vi "Main_ProducerConsumer.vi"() -> ()   [LabVIEW 2014]
doc: "Use this template to build a producer/consumer design pattern. Use this template when you need to execute a process, such as data analysis, when a data source, such as a triggered acquisition, produces data at an uneven rate and you need to execute the process when the data becomes available."
panel:
  in  "WebApp Sensor Data":T1
  in  "WebApp Plug Data":T2
  in  "WebApp Sensors":T3
  in  "WebApp Plugs":T4
  out "plug5option":string
  out "plug4option":string
  out "plug3option":string
  out "plug2option":string
  out "plug1option":string
  out "humidity":string
  out "luminosity":string
  out "temperature":string
  out "Outlet5_Output":bool
  in  "Outlet5_Input":bool
  out "Outlet4_Output":bool
  in  "Outlet4_Input":bool
  out "Outlet3_Output":bool
  in  "Outlet3_Input":bool
  out "Outlet2_Output":bool
  in  "Outlet2_Input":bool
  out "Outlet1_Output":bool
  in  "Outlet1_Input":bool
  in  "Outlet5_Refnum":refnum<k21>="ni.var.psp://Deepak-PC/Shared Variable Library Master/Outlet5"
  in  "Outlet4_Refnum":refnum<k21>="ni.var.psp://Deepak-PC/Shared Variable Library Master/Outlet4"
  in  "Outlet3_Refnum":refnum<k21>="ni.var.psp://Deepak-PC/Shared Variable Library Master/Outlet3"
  in  "Outlet2_Refnum":refnum<k21>="ni.var.psp://Deepak-PC/Shared Variable Library Master/Outlet2"
  in  "Outlet1_Refnum":refnum<k21>="ni.var.psp://Deepak-PC/Shared Variable Library Master/Outlet1"
  in  "stop":bool
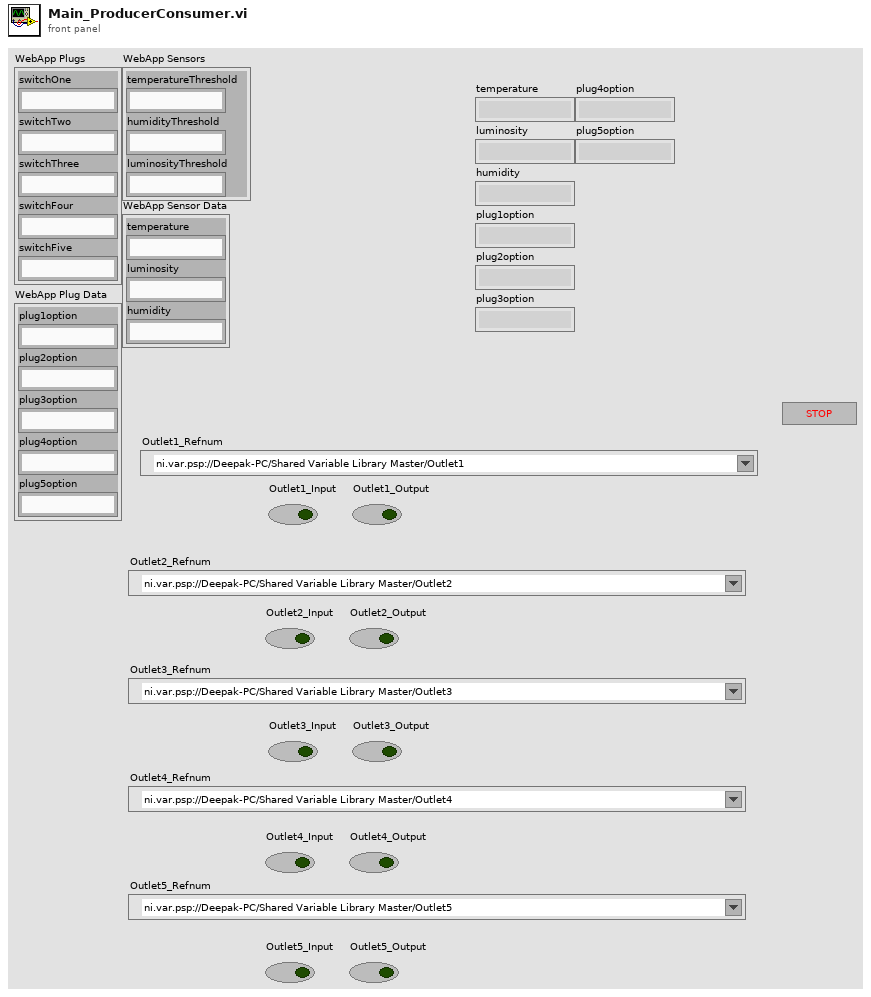
[diagram p1: front panel]
types:
  T1 = cluster{"temperature":string, "luminosity":string, "humidity":string}
  T2 = cluster{"plug1option":string, "plug2option":string, "plug3option":string, "plug4option":string, "plug5option":string}
  T3 = cluster{"temperatureThreshold":string, "humidityThreshold":string, "luminosityThreshold":string}
  T4 = cluster{"switchOne":string, "switchTwo":string, "switchThree":string, "switchFour":string, "switchFive":string}
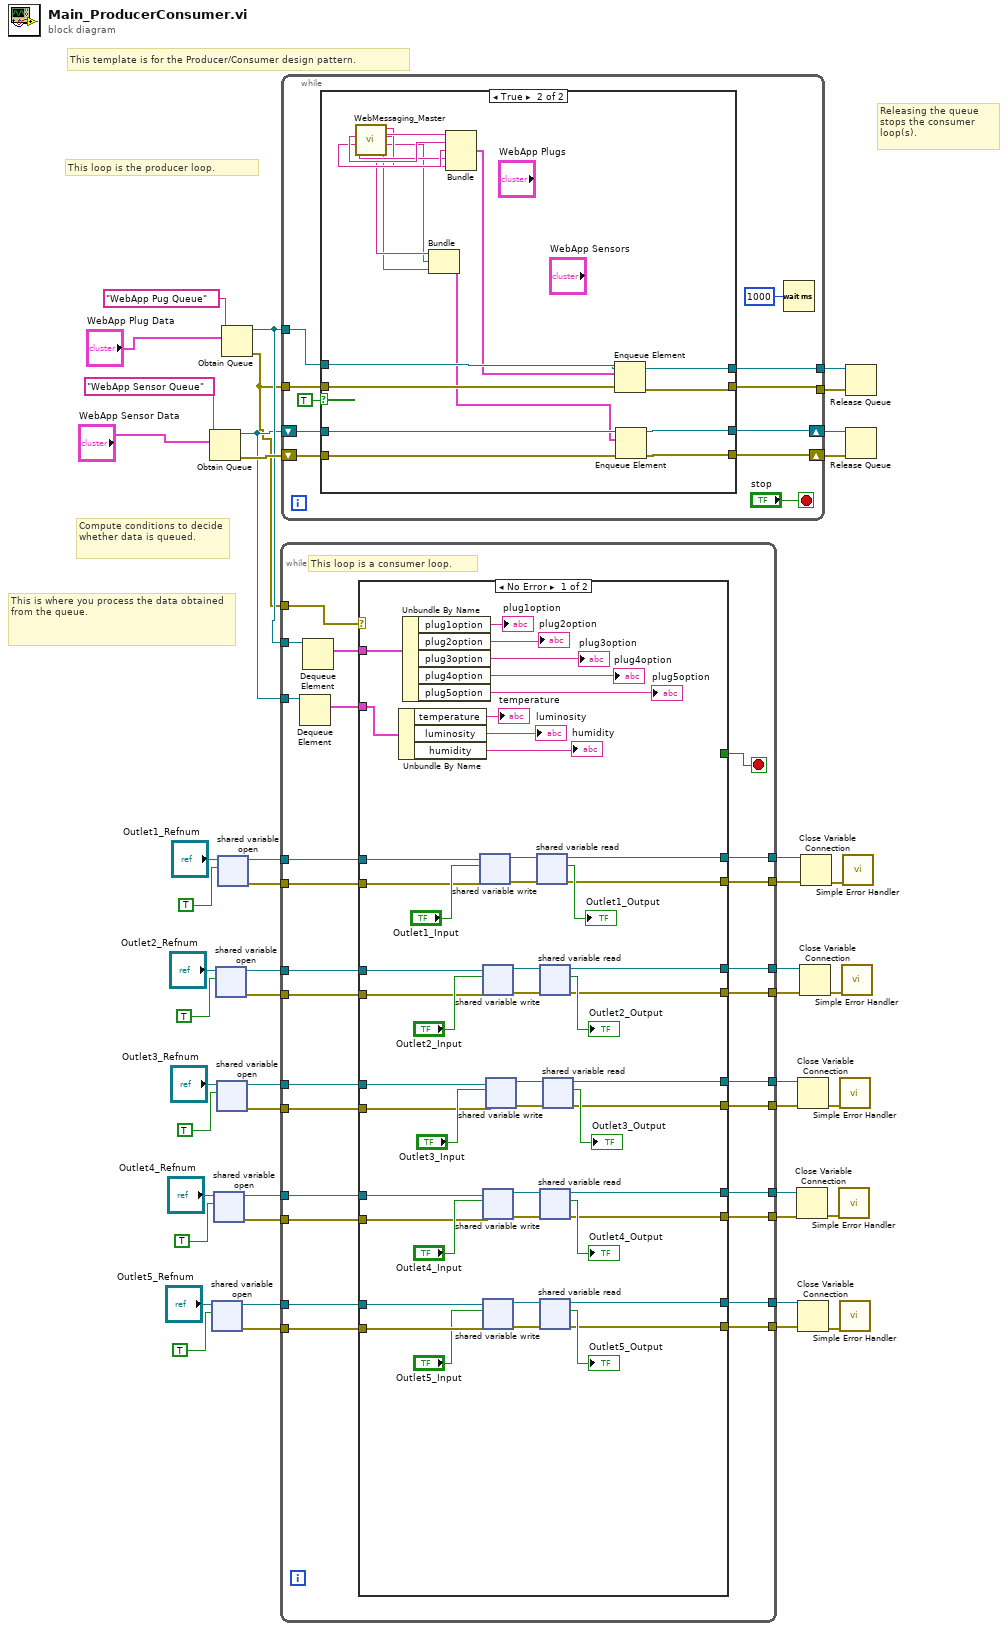
[diagram p0: block diagram]
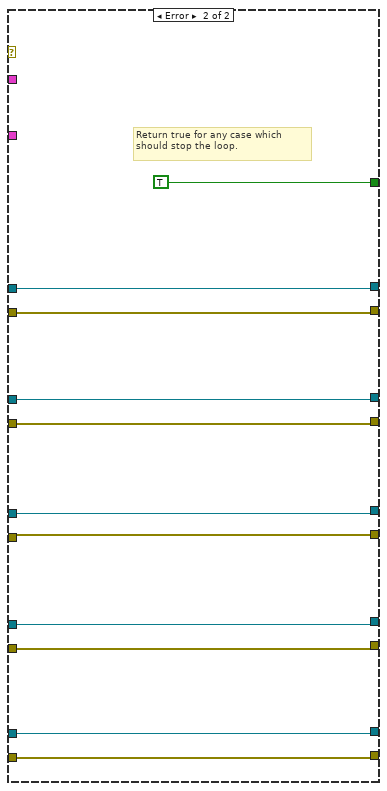
[diagram p2: hidden frame]
diagram:
  # "This is where you process the data obtained from the queue."
  # "This loop is the producer loop."
  # "Compute conditions to decide whether data is queued."
  # "Releasing the queue stops the consumer loop(s)."
  # "This template is for the Producer/Consumer design pattern."
  n1 = Obtain Queue(name (unnamed)="WebApp Sensor Queue", element data type="WebApp Sensor Data") -> (queue out=w37:refnum<queue>, error out=w47:errorcluster)  [unwired: 3 in, 1 out]
  n2 = shared-variable-open("Outlet5_Refnum", TRUE) -> (w5:refnum<k21>, w3:errorcluster)  [unwired: 2 in]
  n3 = shared-variable-open("Outlet4_Refnum", TRUE) -> (w9:refnum<k21>, w7:errorcluster)  [unwired: 2 in]
  n4 = shared-variable-open("Outlet2_Refnum", TRUE) -> (w17:refnum<k21>, w15:errorcluster)  [unwired: 2 in]
  n5 = shared-variable-open("Outlet3_Refnum", TRUE) -> (w13:refnum<k21>, w11:errorcluster)  [unwired: 2 in]
  n6 = shared-variable-open("Outlet1_Refnum", TRUE) -> (w21:refnum<k21>, w19:errorcluster)  [unwired: 2 in]
  n7 = Obtain Queue(name (unnamed)="WebApp Pug Queue", element data type="WebApp Plug Data") -> (queue out=w38:refnum<queue>, error out=w1:errorcluster)  [unwired: 3 in, 1 out]
  n8 = while {
    tunnel: w38 -> [w72]
    tunnel: w37 -> [w71]
    tunnel: w21 -> [w68]
    tunnel: [w67] -> w20
    tunnel: w19 -> [w66]
    tunnel: [w65] -> w18
    tunnel: w17 -> [w64]
    tunnel: [w63] -> w16
    tunnel: w15 -> [w62]
    tunnel: [w61] -> w14
    tunnel: w13 -> [w60]
    tunnel: [w59] -> w12
    tunnel: w11 -> [w58]
    tunnel: [w57] -> w10
    tunnel: w9 -> [w56]
    tunnel: [w55] -> w8
    tunnel: w7 -> [w54]
    tunnel: [w53] -> w6
    tunnel: w5 -> [w52]
    tunnel: [w51] -> w4
    tunnel: w3 -> [w50]
    tunnel: [w49] -> w2
    tunnel: w1 -> [w48]
    stop <- w73 stop-if-true
    # "This loop is a consumer loop."
    n9 = Dequeue Element(queue=w71) -> (element=w69:T1)  [unwired: 2 in, 3 out]
    n10 = Dequeue Element(queue=w72) -> (element=w70:T2)  [unwired: 2 in, 3 out]
    n11 = case shown="No Error" w48 {
      tunnel: [_ TRUE] -> w73
      tunnel: w70 -> [w83 _]
      tunnel: w69 -> [w82 _]
      tunnel: w68 -> [w104 w133]
      tunnel: [w103 w133] -> w67
      tunnel: w66 -> [w102 w132]
      tunnel: [w101 w132] -> w65
      tunnel: w64 -> [w100 w131]
      tunnel: [w99 w131] -> w63
      tunnel: w62 -> [w98 w130]
      tunnel: [w97 w130] -> w61
      tunnel: w60 -> [w96 w129]
      tunnel: [w95 w129] -> w59
      tunnel: w58 -> [w94 w128]
      tunnel: [w93 w128] -> w57
      tunnel: w56 -> [w92 w127]
      tunnel: [w91 w127] -> w55
      tunnel: w54 -> [w90 w126]
      tunnel: [w89 w126] -> w53
      tunnel: w52 -> [w88 w125]
      tunnel: [w87 w125] -> w51
      tunnel: w50 -> [w86 w124]
      tunnel: [w85 w124] -> w49
      frame No Error {
        n12 = Unbundle By Name(w82) -> ("temperature"=→"temperature":string, "luminosity"=→"luminosity":string, "humidity"=→"humidity":string)
        n13 = Unbundle By Name(w83) -> ("plug1option"=→"plug1option":string, "plug2option"=→"plug2option":string, "plug3option"=→"plug3option":string, "plug4option"=→"plug4option":string, "plug5option"=→"plug5option":string)
        n14 = shared-variable-write(w104, w102, "Outlet1_Input") -> (w123:refnum<k21>, w122:errorcluster)
        n15 = shared-variable-write(w100, w98, "Outlet2_Input") -> (w116:refnum<k21>, w117:errorcluster)
        n16 = shared-variable-write(w92, w90, "Outlet4_Input") -> (w108:refnum<k21>, w109:errorcluster)
        n17 = shared-variable-write(w88, w86, "Outlet5_Input") -> (w107:refnum<k21>, w106:errorcluster)
        n18 = shared-variable-write(w96, w94, "Outlet3_Input") -> (w115:refnum<k21>, w114:errorcluster)
        n19 = shared-variable-read(w123, w122) -> (w103:refnum<k21>, w101:errorcluster, →"Outlet1_Output":bool)  [unwired: 1 out]
        n20 = shared-variable-read(w116, w117) -> (w99:refnum<k21>, w97:errorcluster, →"Outlet2_Output":bool)  [unwired: 1 out]
        n21 = shared-variable-read(w108, w109) -> (w91:refnum<k21>, w89:errorcluster, →"Outlet4_Output":bool)  [unwired: 1 out]
        n22 = shared-variable-read(w107, w106) -> (w87:refnum<k21>, w85:errorcluster, →"Outlet5_Output":bool)  [unwired: 1 out]
        n23 = shared-variable-read(w115, w114) -> (w95:refnum<k21>, w93:errorcluster, →"Outlet3_Output":bool)  [unwired: 1 out]
      }
      frame Error {
        # "Return true for any case which should stop the loop."
      }
    }
  }
  n24 = while {
    shift-right: [w141] -> w45
    shift-left: w47 -> [w142]
    shift-right: [w143] -> w46
    shift-left: w37 -> [w144]
    tunnel: [w138] -> w40
    tunnel: w1 -> [w137]
    tunnel: w38 -> [w136]
    tunnel: [w135] -> w39
    stop <- "stop" stop-if-true
    n25 = case shown="True" TRUE ("Case Constant\n(See Context Help)") {
      tunnel: w144 -> [w149 w167]
      tunnel: [w149 w166] -> w143
      tunnel: w142 -> [w148 w165]
      tunnel: [w148 w164] -> w141
      tunnel: [w147 w162] -> w138
      tunnel: w137 -> [w147 w163]
      tunnel: w136 -> [w146 w161]
      tunnel: [w146 w160] -> w135
      frame False {
      }
      frame True {
        n26 = call "WebMessaging_Master.vi"() -> ("luminosityThreshold"=w151:string, "humidityThreshold"=w152:string, "temperatureThreshold"=w153:string, "switchFive"=w155:string, "switchFour"=w156:string, "switchThree"=w157:string, "switchTwo"=w158:string, "switchOne"=w159:string)  [unwired: 4 in]
        n27 = Bundle("temperatureThreshold"=w153, "humidityThreshold"=w152, "luminosityThreshold"=w151) -> (w150:T3)  [unwired: 1 in]
        n28 = Bundle("switchOne"=w159, "switchTwo"=w158, "switchThree"=w157, "switchFour"=w156, "switchFive"=w155) -> (w154:T4)  [unwired: 1 in]
        n29 = Enqueue Element(queue=w161, element=w154, error in (no error)=w163) -> (queue out=w160:refnum<queue>, error out=w162:errorcluster)  [unwired: 1 in, 1 out]
        n30 = Enqueue Element(queue=w167, element=w150, error in (no error)=w165) -> (queue out=w166:refnum<queue>, error out=w164:errorcluster)  [unwired: 1 in, 1 out]
      }
    }
    n31 = Wait (ms)(milliseconds to wait=u32 1000) -> ()  [unwired: 1 out]
  }
  n32 = Close Variable Connection(8:w6, 11:w8) -> (0:w24:errorcluster)
  n33 = Close Variable Connection(8:w10, 11:w12) -> (0:w23:errorcluster)
  n34 = Close Variable Connection(8:w2, 11:w4) -> (0:w22:errorcluster)
  n35 = Close Variable Connection(8:w14, 11:w16) -> (0:w25:errorcluster)
  n36 = Close Variable Connection(8:w18, 11:w20) -> (0:w26:errorcluster)
  n37 = call <vilib>:"Simple Error Handler.vi"("error in (no error)"=w24) -> ()  [unwired: 4 in, 5 out]
  n38 = call <vilib>:"Simple Error Handler.vi"("error in (no error)"=w23) -> ()  [unwired: 4 in, 5 out]
  n39 = call <vilib>:"Simple Error Handler.vi"("error in (no error)"=w22) -> ()  [unwired: 4 in, 5 out]
  n40 = call <vilib>:"Simple Error Handler.vi"("error in (no error)"=w25) -> ()  [unwired: 4 in, 5 out]
  n41 = call <vilib>:"Simple Error Handler.vi"("error in (no error)"=w26) -> ()  [unwired: 4 in, 5 out]
  n42 = Release Queue(queue=w39, error in (no error)=w40) -> ()  [unwired: 1 in, 3 out]
  n43 = Release Queue(queue=w46, error in (no error)=w45) -> ()  [unwired: 1 in, 3 out]
